vi "WinConditionOutside.vi"(8 "error in (no error)":errorcluster, 11 "Gameplay Data":T2) -> (0 "error out":errorcluster, 1 "LineIndices":i8[](array[numeric]), 2 "Winner":T1, 3 "End?":bool)   [LabVIEW 2020]
uses:
  controls/Gameplay Data.ctl
  controls/Gameboard Refnums.ctl
  controls/General Refnums.ctl
  controls/Gameboard Data.ctl
  controls/Player.ctl
  controls/PlayerMode.ctl
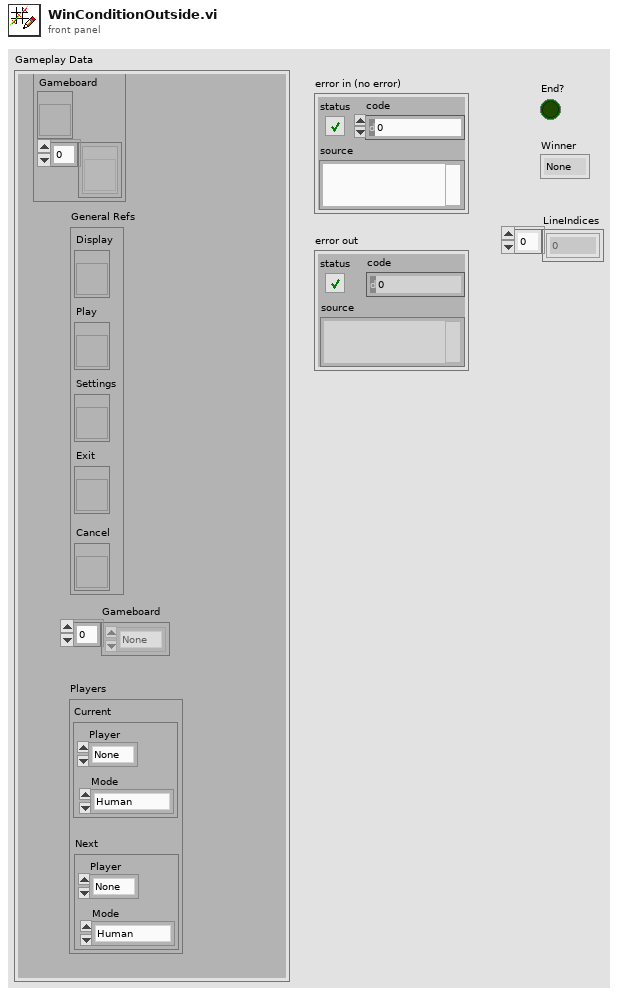
[diagram p1: front panel]
types:
  T1 = typedef "Player.ctl" = enum16{"None", "Player 1", "Player 2"}
  T2 = typedef "Gameplay Data.ctl" = cluster{"Gameboard Refs":T3, "General Refs":T4, "Gameboard":T5, "Players":cluster{"Current":cluster{"Player":T1, "Mode":T6}, "Next":cluster{"Player":T1, "Mode":T6}}}
  T3 = typedef "Gameboard Refnums.ctl" = cluster{"Gameboard":refnum<vi>, "Button Refs":refnum<vi>[]}
  T4 = typedef "General Refnums.ctl" = cluster{"Display":refnum<vi>, "Play":refnum<vi>, "Settings":refnum<vi>, "Exit":refnum<vi>, "Cancel":refnum<vi>}
  T5 = typedef "Gameboard Data.ctl" = enum16{"None", "Player 1", "Player 2"}[]
  T6 = typedef "PlayerMode.ctl" = enum16{"Human", "BotRand", "BotHeur1"}
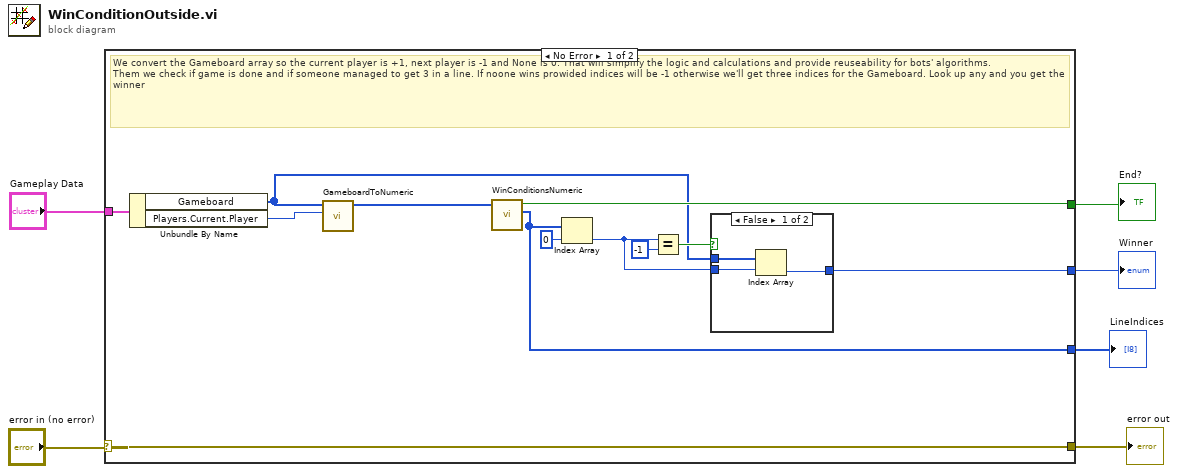
[diagram p0: block diagram]
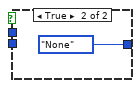
[diagram p2: hidden frame]
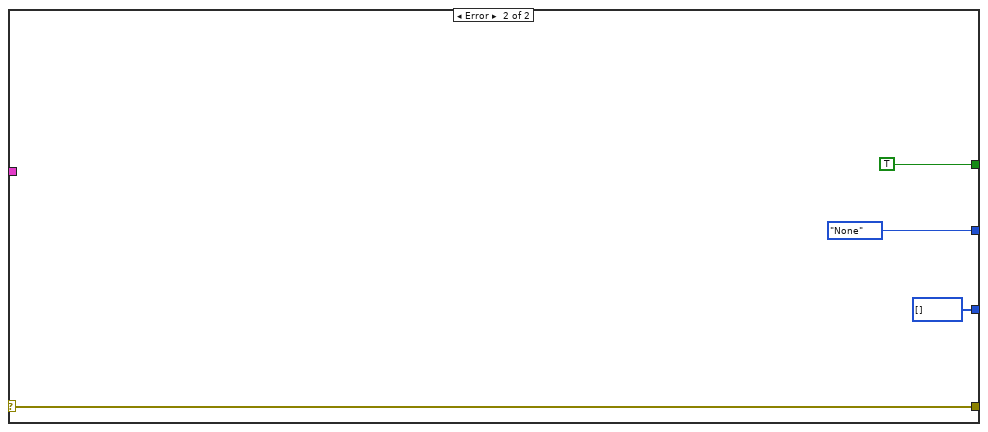
[diagram p3: hidden frame]
diagram:
  n1 = case shown="No Error" "error in (no error)" {
    selector: "error in (no error)" -> [w18 w26]
    tunnel: [w18 w26] -> w5
    tunnel: [w16 TRUE ("End?")] -> w4
    tunnel: [w12 Player."None" ("Winner")] -> w3
    tunnel: "Gameplay Data" -> [w17 _]
    tunnel: [w8 i8[] [] ("LineIndices")] -> w1
    frame No Error {
      # "We convert the Gameboard array so the current player is +1, next player is -1 and None is 0. That will simplify the logic and calculations and provide reuseability for bots' algorithms.\nThem we check if game is done and if someone managed to get 3 in a line. If noone wins prowided indices will be -1 otherwise we'll get three indices for the Gameboard. Look up any and you get the winner"
      n2 = Unbundle By Name(w17) -> ("Gameboard"=w7:T5, "Players.Current.Player"=w9:T1)
      n3 = call "GameboardToNumeric.vi"("CurrentPlayer"=w9, "Gameboard"=w7) -> ("NumericGameboard"=w10:i8[])  [unwired: 9 in]
      n4 = call "WinConditionsNumeric.vi"("NumericGameboard"=w10) -> ("LineIndices"=w8:i8[], "End?"=w16:bool)  [unwired: 9 in]
      n5 = Index Array(array=w8, index=0) -> (element=w11:i8)
      n6 = Equal?(x=w11, y=i8 -1) -> (x = y?=w13:bool)
      n7 = case shown="False" w13 {
        tunnel: [w20 Player."None" ("Winner")] -> w12
        tunnel: w11 -> [w21 _]
        tunnel: w7 -> [w19 _]
        frame False {
          n8 = Index Array(array=w19, index=w21) -> (element=w20:enum16{"None", "Player 1", "Player 2"})
        }
        frame True {
        }
      }
    }
    frame Error {
    }
  }
  "error out" <- w5
  "End?" <- w4
  "Winner" <- w3
  "LineIndices" <- w1
